vi "Utility_Sort Colors 1D Array.vi"(8 "Error":errorcluster, 11 "Colors":u32[](array[colorbox])) -> (0 "Error Out":errorcluster, 2 "Count Out":u32[](array[numeric]), 3 "Sorted By Quantity Out":u32[](array[colorbox]))   [LabVIEW 2009]
doc: "Sorts the color array by size"
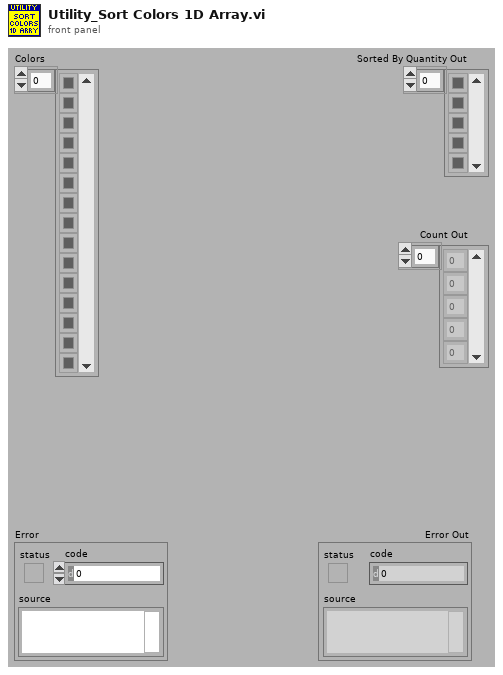
[diagram p1: front panel]
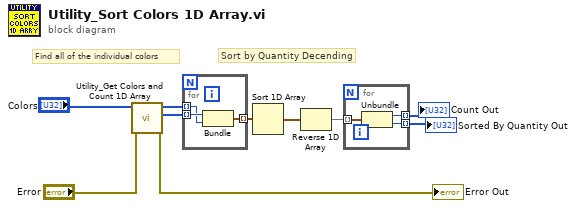
[diagram p0: block diagram]
diagram:
  # "Sort by Quantity Decending"
  # "Find all of the individual colors"
  n1 = call "Utility_Get Colors and Count 1D Array.vi"("Error"="Error", "Color Array"="Colors") -> ("Error Out"=→"Error Out":errorcluster, "Count Out"=w5:u32[], "Color List Out"=w6:u32[])  [unwired: 7 in]
  n2 = for {
    tunnel: w5 -> [w13] mode=indexing
    tunnel: w6 -> [w12] mode=indexing
    tunnel: [w11] -> w10 mode=indexing
    n3 = Bundle(w13, w12) -> (w11:cluster{u32, u32})  [unwired: 1 in]
  }
  n4 = Sort 1D Array(array=w10) -> (sorted array=w9:cluster{u32, u32}[])
  n5 = Reverse 1D Array(array=w9) -> (reversed array=w7:cluster{u32, u32}[])
  n6 = for {
    tunnel: w7 -> [w16] mode=indexing
    tunnel: [w15] -> w8 mode=indexing
    tunnel: [w14] -> w1 mode=indexing
    n7 = Unbundle(w16) -> (w14:u32, w15:u32)
  }
  "Sorted By Quantity Out" <- w8
  "Count Out" <- w1
